vi "Add Topic.vi"(8 "error in (no error)":errorcluster, 9 "Topic Enqueuer":refnum<class "Message Enqueuer.lvclass">, 10 "Topic Object":refnum<class "Topic.lvclass">, 11 "TopicLookupTable":refnum<data-value>) -> (0 "error out":errorcluster, 2 "Topic Replaced?":bool, 3 "TopicLookupTable":refnum<data-value>)   [LabVIEW 2018, in "MVA Framework.lvlib" / "Mediator.lvlib" / "TopicLookupTable.lvclass"]
doc: "<License>\nCopyright © 2017 Composed Systems, LLC | All rights reserved\nwww.composed.io\n\nAuthor: Ethan Stern <ethan.stern@composed.io>\n\nThis software is provided \"AS IS\" WITHOUT WARRANTIES, either express or implied, AND IS FOR EDUCATIONAL PURPOSES ONLY.\n</License>"
uses:
  TopicLookupTable.lvclass
  Topic/Topic.lvclass
  <vilib>/ErrorRing/Error Ring.xnode
  <vilib>/ActorFramework/Message Enqueuer/Message Enqueuer.lvclass
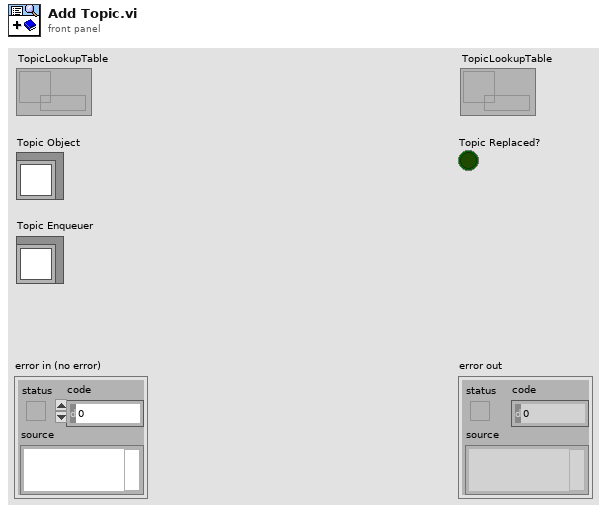
[diagram p1: front panel]
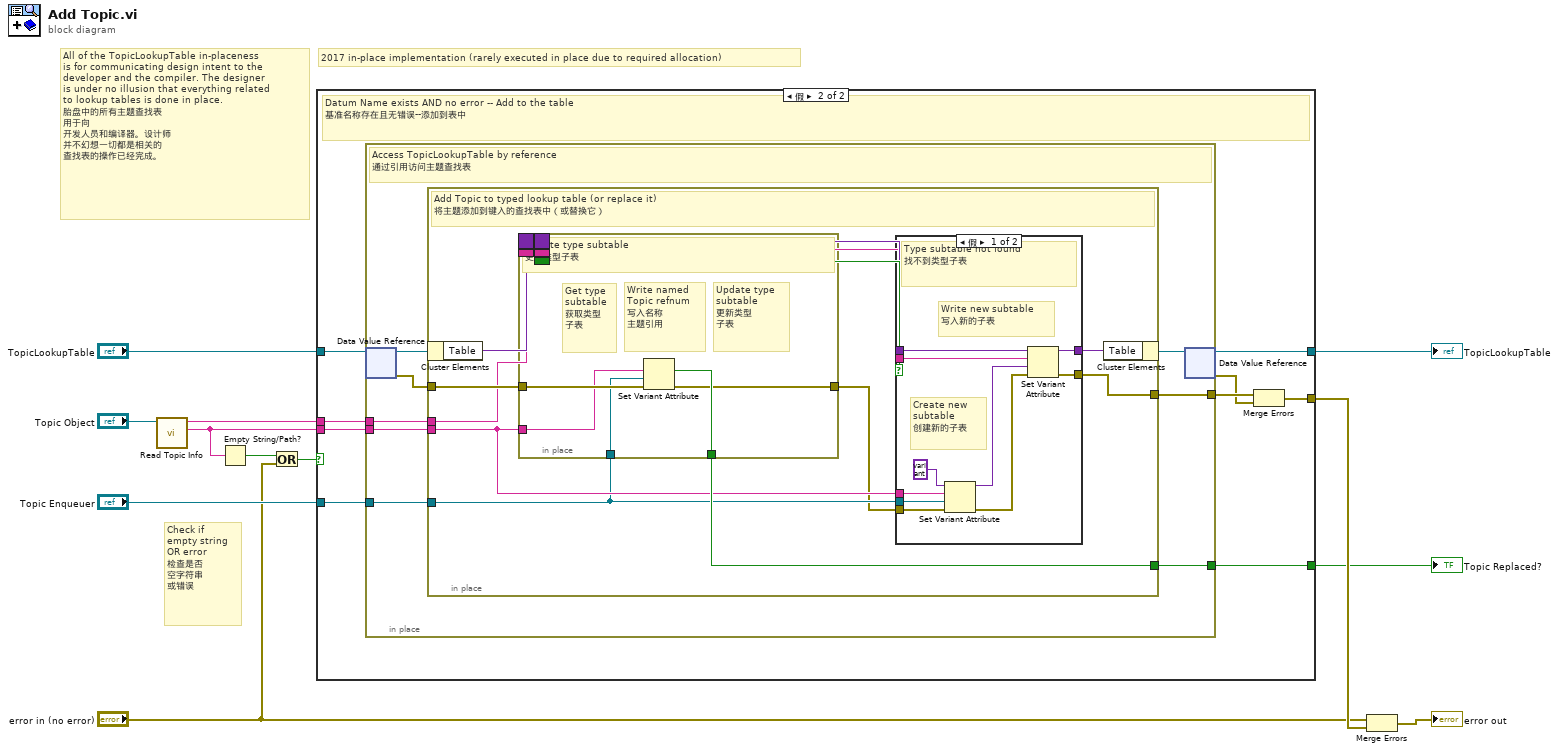
[diagram p0: block diagram]
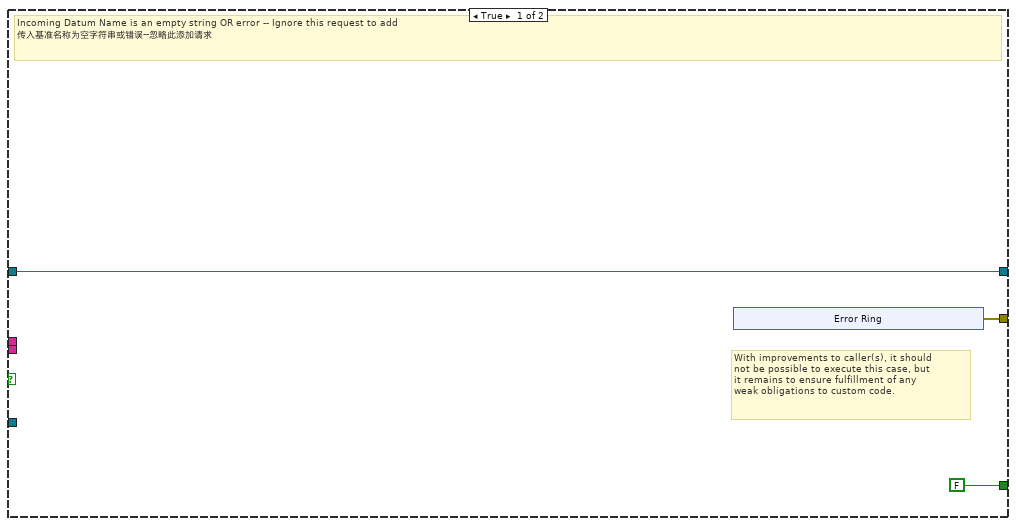
[diagram p2: hidden frame]
diagram:
  # "2017 in-place implementation (rarely executed in place due to required allocation)"
  # "Check if\nempty string\nOR error\n检查是否\n空字符串\n或错误"
  # "All of the TopicLookupTable in-placeness\nis for communicating design intent to the\ndeveloper and the compiler. The designer\nis under no illusion that everything related\nto lookup tables is done in place.\n胎盘中的所有主题查找表\n用于向\n开发人员和编译器。设计师\n并不幻想一切都是相关的\n查找表的操作已经完成。"
  n1 = call "Read Topic Info.vi"("Topic in"="Topic Object") -> ("Name"=w2:string, "Type"=w6:string)  [unwired: 7 in, 2 out]
  n2 = Empty String/Path?(string/path=w2) -> (empty?=w3:bool)
  n3 = Or(x=w3, y="error in (no error)") -> (x .or. y?=w1:bool)
  n4 = case shown="假" w1 {
    tunnel: "TopicLookupTable" -> [w13 w22]
    tunnel: [w14 w21] -> w10
    tunnel: [FALSE ("replaced") w25] -> w9
    tunnel: "Topic Enqueuer" -> [_ w24]
    tunnel: w6 -> [_ w23]
    tunnel: [w13 w20] -> w5
    tunnel: w2 -> [_ w19]
    frame True {
      # "With improvements to caller(s), it should\nnot be possible to execute this case, but\nit remains to ensure fulfillment of any\nweak obligations to custom code."
      # "Incoming Datum Name is an empty string OR error -- Ignore this request to add\n传入基准名称为空字符串或错误--忽略此添加请求"
      n5 = xnode "Error Ring"() -> ("错误输出"=w14:errorcluster)
    }
    frame False {
      # "Datum Name exists AND no error -- Add to the table\n基准名称存在且无错误--添加到表中"
      n6 = in-place {
        in-place-border: [w33] -> w25
        in-place-border: w24 -> [w32]
        in-place-border: w23 -> [w31]
        in-place-border: w19 -> [w30]
        in-place-border: [w26] -> w18
        # "Access TopicLookupTable by reference\n通过引用访问主题查找表"
        n7 = in-place-dvr #1(w22) -> (w29:refnum<class "TopicLookupTable.lvclass">, w27:errorcluster)
        n8 = in-place {
          in-place-border: [w44] -> w33
          in-place-border: w32 -> [w36]
          in-place-border: w31 -> [w42]
          in-place-border: w30 -> [w37]
          in-place-border: w27 -> [w45]
          in-place-border: [w34] -> w26
          # "Add Topic to typed lookup table (or replace it)\n将主题添加到键入的查找表中（或替换它）"
          n9 = in-place-cluster #2(w29) -> ("Table"=w43:variant)
          n10 = in-place {
            in-place-border: [w50] -> w44
            in-place-border: w36 -> [w47]
            in-place-border: w37 -> [w48]
            border: w43 -> [_]
            border: w42 -> [_]
            border: [_] -> w40
            border: [_] -> w38
            border: [_] -> w41
            in-place-border: w45 -> [w52]
            in-place-border: [w46] -> w35
            # "Write named\nTopic refnum\n写入名称\n主题引用"
            # "Update type\nsubtable\n更新类型\n子表"
            # "Get type\nsubtable\n获取类型\n子表"
            # "Update type subtable\n更新类型子表"
            n11 = Set Variant Attribute(Variant=w49, name=w48, value=w47, error in=w52) -> (Variant out=w51:variant, replaced=w50:bool, error out=w46:errorcluster)
          }
          n12 = case shown="假" w41 {
            tunnel: w40 -> [w62 w64]
            tunnel: [w61 w64] -> w39
            tunnel: w38 -> [w60 _]
            tunnel: w37 -> [w59 _]
            tunnel: w36 -> [w58 _]
            tunnel: w35 -> [w54 w63]
            tunnel: [w53 w63] -> w34
            frame False {
              # "Write new subtable\n写入新的子表"
              # "Create new\nsubtable\n创建新的子表"
              # "Type subtable not found\n找不到类型子表"
              n13 = Set Variant Attribute(Variant=variant ("variant"), name=w59, value=w58, error in=w54) -> (Variant out=w57:variant, error out=w55:errorcluster)  [unwired: 1 out]
              n14 = Set Variant Attribute(Variant=w62, name=w60, value=w57, error in=w55) -> (Variant out=w61:variant, error out=w53:errorcluster)  [unwired: 1 out]
            }
            frame True {
              # "Subtable updated okay"
            }
          }
          n15 = in-place-cluster #2("Table"=w39) -> (w28:refnum<class "TopicLookupTable.lvclass">)
        }
        n16 = in-place-dvr #1(w28) -> (w20:refnum<data-value>, w17:errorcluster)
      }
      n17 = Merge Errors(w18, w17) -> (w21:errorcluster)
    }
  }
  "Topic Replaced?" <- w9
  "TopicLookupTable" <- w5
  n18 = Merge Errors("error in (no error)", w10) -> (→"error out":errorcluster)
